vi "json.replace.vi"(8 "error in":errorcluster, 9 "Object To Update":string, 10 "JSON in":string, 11 "timestampMetadata in":refnum<class "timestampMetadata.lvclass">) -> (0 "error out":errorcluster, 2 "JSON out":string, 3 "timestampMetadata out":refnum<class "timestampMetadata.lvclass">)   [LabVIEW 2018, in "timestampMetadata.lvclass"]
uses:
  timestampMetadata.lvclass
  <vilib>/JDP Science/JSONtext/JSONtext.lvlib
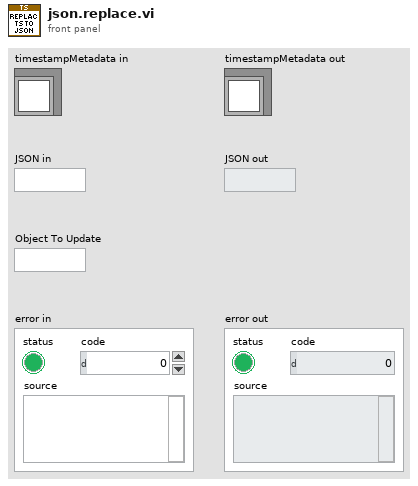
[diagram p1: front panel]
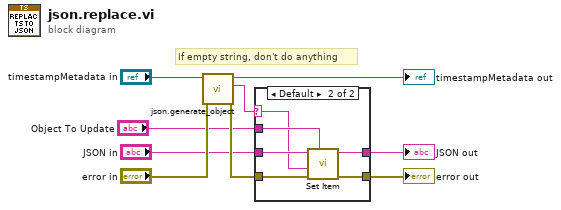
[diagram p0: block diagram]
diagram:
  # "If empty string, don't do anything"
  n1 = call-dynamic "json.generate_object.vi"("error in"="error in", "timestampMetadata in"="timestampMetadata in") -> ("error out"=w6:errorcluster, "JSON Object"=w7:string, "timestampMetadata out"=→"timestampMetadata out":refnum<class "timestampMetadata.lvclass">)  [unwired: 7 in]
  n2 = case shown="Default" w7 {
    selector: w7 -> [_ w14]
    tunnel: "JSON in" -> [w11 w17]
    tunnel: w6 -> [w10 w13]
    tunnel: [w11 w15] -> w5
    tunnel: "Object To Update" -> [_ w16]
    tunnel: [w10 w12] -> w4
    frame "" {
    }
    frame Default {
      n3 = call <vilib>:"Set Item.vi"("$Path or Item Name"=w16, "error in (no error)"=w13, "JSON to Insert"=w14, "JSON"=w17) -> ("error out"=w12:errorcluster, "<JSON>"=w15:string)  [unwired: 4 in, 1 out]
    }
  }
  "error out" <- w4
  "JSON out" <- w5
